vi "Odbiór UDP z SbRIO.vi"(5 "Queue in":refnum<queue>, 7 "error in queue":errorcluster, 8 "error in udp (no error)":errorcluster, 11 "port":refnum<k16>) -> (0 "error out udp":errorcluster, 1 "error out variant":errorcluster, 3 "UDP Network Connection out":refnum<k16>)   [LabVIEW 2014]
uses:
  Program Files (x86)/National Instruments/LabVIEW 2014/examples/Design Patterns/Queued Message Handler/support/QMH Fundamentals - Message Cluster.ctl
  CANFrameControl.ctl
types:
  T1 = typedef "QMH Fundamentals - Message Cluster.ctl" = cluster{"Message":string, "Message Data":variant}
  T2 = typedef "CANFrameControl.ctl" = cluster{"identifier":u32, "extended?":bool, "type":u8, "payload":u8[]}
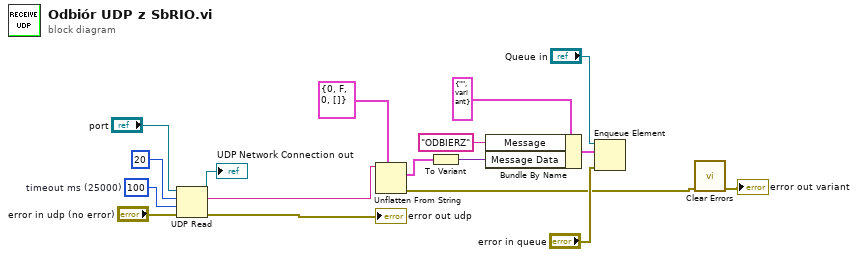
[diagram p0: block diagram]
diagram:
  w17 = 100  # timeout ms (25000)
  n1 = UDP Read(connection ID="port", max size (548)=20, timeout ms (25000)=w17, 8:"error in udp (no error)") -> (data out=w5:string, error out=→"error out udp":errorcluster, 3:→"UDP Network Connection out":refnum<k16>)  [unwired: 2 out]
  n2 = Unflatten From String(type=T2 {"identifier"=0, "extended?"=FALSE, "type"=0, "payload"=[]} ("CAN frame 3"), binary string=w5) -> (value=w11:T2, error out=w2:errorcluster)  [unwired: 3 in, 1 out]
  n3 = To Variant(anything=w11) -> (Variant=w10:variant)
  n4 = Bundle By Name(cluster=T1 {"Message"="", "Message Data"=variant} ("Message Cluster"), "Message"="ODBIERZ", "Message Data"=w10) -> (w14:T1)
  n5 = Enqueue Element(queue="Queue in", element=w14, error in (no error)="error in queue") -> ()  [unwired: 1 in, 3 out]
  n6 = call <vilib>:"Clear Errors.vi"("error in (no error)"=w2) -> ("error out"=→"error out variant":errorcluster)  [unwired: 5 in, 1 out]
